vi "Initial Password.vi"(8 "error in (no error)":errorcluster, 11 "Master in":refnum<class "Master.lvclass">) -> (0 "error out":errorcluster, 3 "Master out":refnum<class "Master.lvclass">)   [LabVIEW 2014, in "Master.lvclass"]
uses:
  Master/Master.lvclass
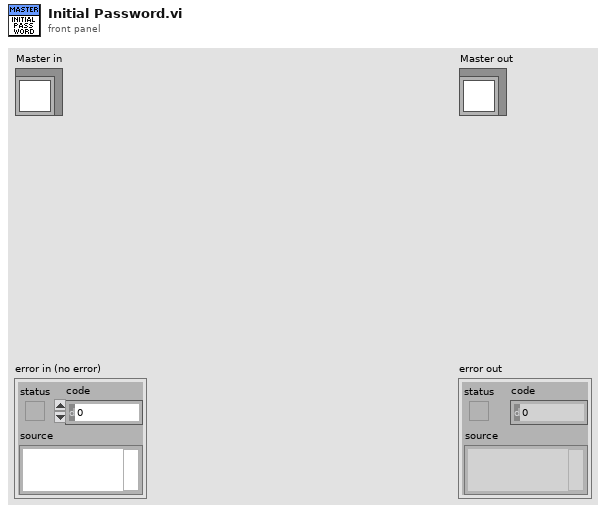
[diagram p1: front panel]
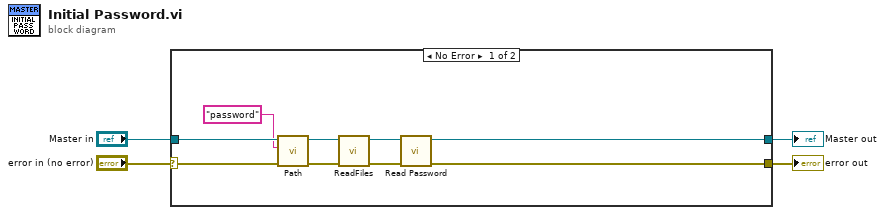
[diagram p0: block diagram]
diagram:
  n1 = case shown="No Error" "error in (no error)" {
    selector: "error in (no error)" -> [w11 w15]
    tunnel: [w8 w15] -> w3
    tunnel: [w7 w14] -> w1
    tunnel: "Master in" -> [w13 w14]
    frame No Error {
      n2 = call-dynamic "Path.vi"("error in (no error)"=w11, "pathname"="password", "Master in"=w13) -> ("error out"=w10:errorcluster, "Master out"=w12:refnum<class "Master.lvclass">)  [unwired: 7 in]
      n3 = call-dynamic "ReadFiles.vi"("error in (no error)"=w10, "Master in"=w12) -> ("error out"=w5:errorcluster, "Master out"=w6:refnum<class "Master.lvclass">)  [unwired: 8 in]
      n4 = call-dynamic "Read Password.vi"("error in (no error)"=w5, "Master in"=w6) -> ("error out"=w8:errorcluster, "Master out"=w7:refnum<class "Master.lvclass">)  [unwired: 8 in]
    }
    frame Error {
    }
  }
  "error out" <- w3
  "Master out" <- w1
